vi "Revision Query.vi"(8 "error in (no error)":errorcluster, 9 "Device and Axis":string, 11 "VISA resource name":refnum<visa-resource-name>) -> (0 "error out":errorcluster, 1 "Instrument Firmware Revision":string, 2 "Instrument Driver Revision":string, 3 "VISA resource name out":refnum<visa-resource-name>)   [LabVIEW 2015, in "Zaber A Series.lvlib"]
doc: "Queries the firmware version of the controller as well as the revision of the instrument driver. \n\nThis VI requires that the Initialize VI has been called with the same serial port. \n\nRefer to the Readme file for detailed driver information including modification history."
uses:
  Zaber A Series.lvlib
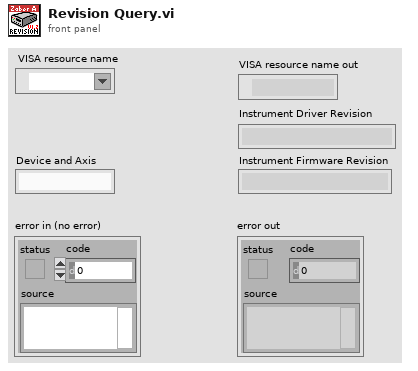
[diagram p1: front panel]
types:
  T1 = cluster{"Major":u16, "Minor":u16, "Fix":u16, "Build":u16}
  T2 = cluster{"Device":string, "Axis":string, "Reply Flag":string, "Status":string, "Warning Flags":string, "Data":string}[]
  T3 = cluster{"Device":string, "Axis":string, "Reply Flag":string, "Status":string, "Warning Flags":string, "Data":string}
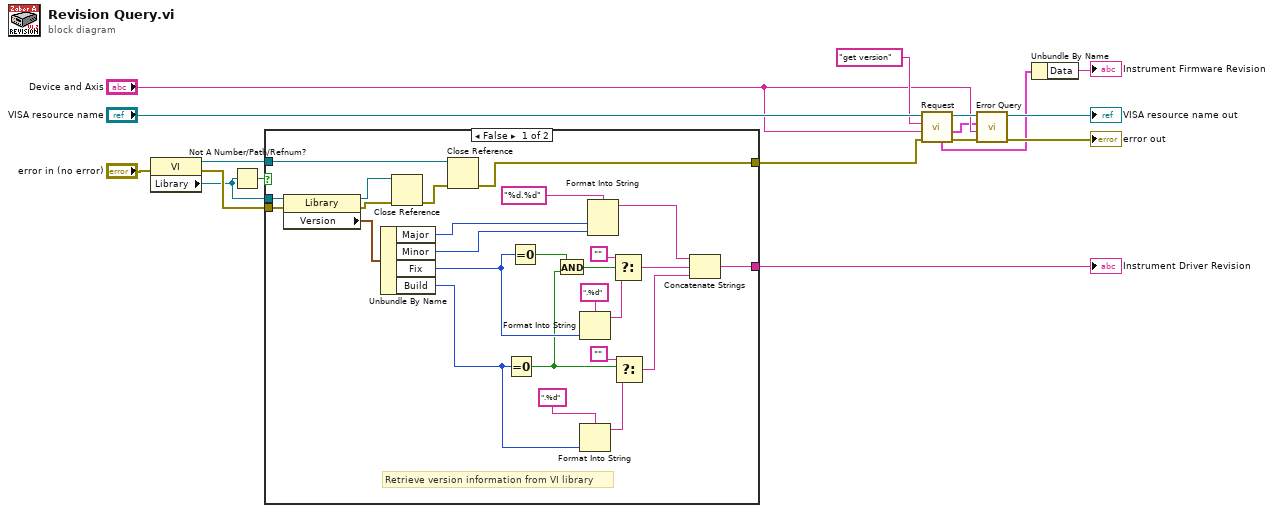
[diagram p0: block diagram]
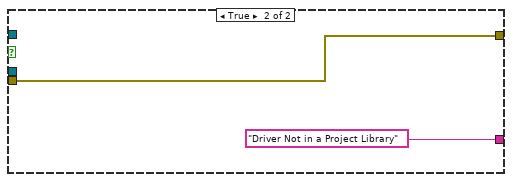
[diagram p2: hidden frame]
diagram:
  n1 = property class="VI"(error in="error in (no error)") -> (reference out=w7:refnum<vi>, error out=w6:errorcluster, "Library"=w5:refnum<vi>)  [unwired: 1 in]
  n2 = Not A Number/Path/Refnum?(number/path/refnum=w5) -> (NaN/Path/Refnum?=w4:bool)
  n3 = case shown="False" w4 {
    tunnel: w7 -> [w40 _]
    tunnel: w6 -> [w25 w45]
    tunnel: [w20 w45] -> w14
    tunnel: [w19 "Driver Not in a Project Library"] -> w15
    tunnel: w5 -> [w18 _]
    frame False {
      # "Retrieve version information from VI library"
      n4 = property class="Library"(reference=w18, error in=w25) -> (reference out=w42:refnum<vi>, error out=w43:errorcluster, "Version"=w39:T1)
      n5 = Unbundle By Name(w39) -> ("Major"=w28:u16, "Minor"=w27:u16, "Fix"=w24:u16, "Build"=w26:u16)
      n6 = Close Reference(reference=w42, error in (no error)=w43) -> (error out=w41:errorcluster)
      n7 = Close Reference(reference=w40, error in (no error)=w41) -> (error out=w20:errorcluster)
      n8 = Equal To 0?(x=w26) -> (x = 0?=w22:bool)
      n9 = Equal To 0?(x=w24) -> (x = 0?=w23:bool)
      n10 = And(x=w23, y=w22) -> (x .and. y?=w21:bool)
      n11 = Format Into String(format string=".%d", w24) -> (resulting string=w36:string)  [unwired: 2 in, 1 out]
      n12 = Format Into String(format string=".%d", w26) -> (resulting string=w32:string)  [unwired: 2 in, 1 out]
      n13 = Format Into String(format string="%d.%d", w28, w27) -> (resulting string=w34:string)  [unwired: 2 in, 1 out]
      n14 = Select(t="", s=w21, f=w36) -> (s? t:f=w33:string)
      n15 = Select(t="", s=w22, f=w32) -> (s? t:f=w29:string)
      n16 = Concatenate Strings(w34, w33, w29) -> (w19:string)
    }
    frame True {
    }
  }
  "Instrument Driver Revision" <- w15
  n17 = call "Request.vi"("error in (no error)"=w14, "Device and Axis"="Device and Axis", "Command String"="get version", "VISA resource name"="VISA resource name") -> ("error out"=w13:errorcluster, "Response Bundle Array"=w2:T2, "VISA resource name out"=w10:refnum<visa-resource-name>, "First Response Bundle"=w1:T3)  [unwired: 2 in, 2 out]
  n18 = call "Error Query.vi"("error in (no error)"=w13, "Device and Axis"="Device and Axis", "Previous Response Bundle Array"=w2, "VISA resource name"=w10) -> ("error out"=→"error out":errorcluster, "VISA resource name out"=→"VISA resource name out":refnum<visa-resource-name>)  [unwired: 4 in, 2 out]
  n19 = Unbundle By Name(w1) -> ("Data"=→"Instrument Firmware Revision":string)
